vi "Untitled 3 (SubVI).vi"(0 "input string":string) -> (1 "btnVal":dbl, 2 "remaining string":string, 3 "potVal":dbl, 5 "Humdity":dbl, 6 "Temperatuur":dbl, 7 "Hic":dbl)   [LabVIEW 2024]
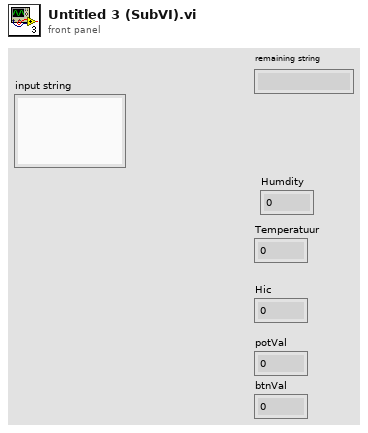
[diagram p1: front panel]
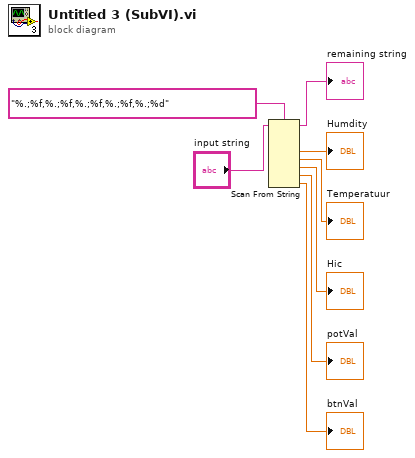
[diagram p0: block diagram]
diagram:
  n1 = Scan From String(format string="%.;%f,%.;%f,%.;%f,%.;%f,%.;%d" ("input string"), input string="input string") -> (remaining string=→"remaining string":string, output 1=→"Humdity":dbl, output 2=→"Temperatuur":dbl, output 3=→"Hic":dbl, output 4=→"potVal":dbl, output 5=→"btnVal":dbl)  [unwired: 7 in, 2 out]
